vi "_API_BINANCE_GET_TickSize.vi"(0 "BinanceAPI in":refnum<class "BinanceAPI_.lvclass">, 5 "TickSize":cluster{"symbol (eg. BTCUSDT)":string}, 11 "error in (no error)":errorcluster) -> (4 "BinanceAPI out":refnum<class "BinanceAPI_.lvclass">, 6 "TickSize":dbl, 15 "error out":errorcluster)   [LabVIEW 2022 SP3, in "BinanceAPI_.lvclass"]
doc: "https://binance-docs.github.io/apidocs/spot/en/#exchange-information\n\nYou must understand what is <B>ticker size</B>"
uses:
  BinanceAPI_.lvclass
  BinanceAPI_.lvclass/BinanceAPI_.ctl
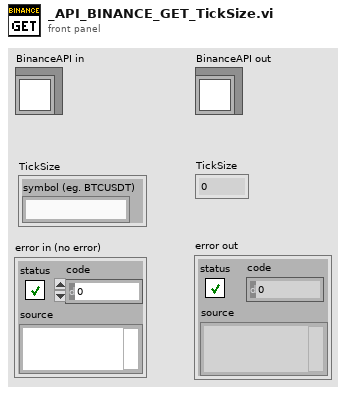
[diagram p1: front panel]
types:
  T1 = enum16{"SPOT", "USDT_FUTURES", "COIN_FUTURES", "VANILLA"}
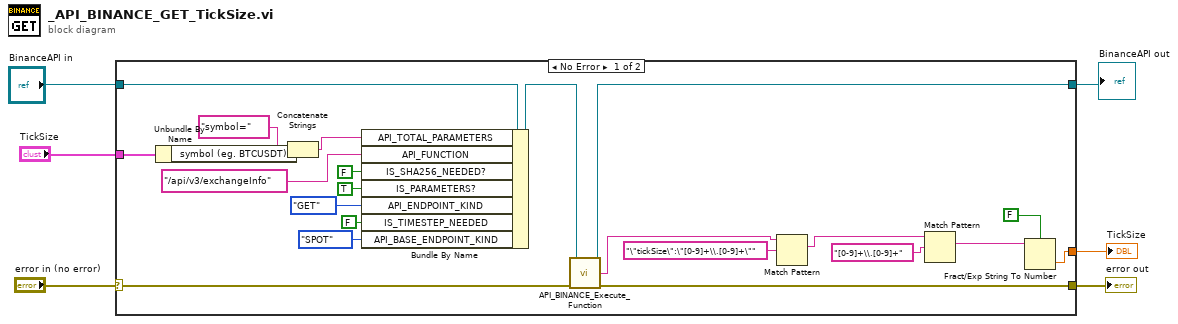
[diagram p0: block diagram]
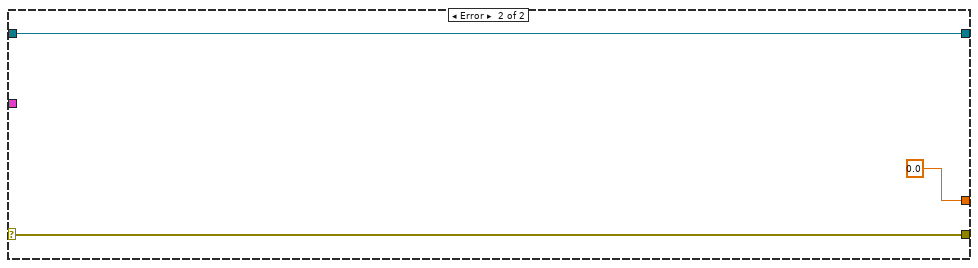
[diagram p2: hidden frame]
diagram:
  n1 = case shown="No Error" "error in (no error)" {
    selector: "error in (no error)" -> [w17 w31]
    tunnel: [w16 w31] -> w5
    tunnel: [w18 w30] -> w2
    tunnel: "BinanceAPI in" -> [w28 w30]
    tunnel: "TickSize" -> [w21 _]
    tunnel: [w9 0.0] -> w4
    frame No Error {
      n2 = Unbundle By Name(w21) -> ("symbol (eg. BTCUSDT)"=w20:string)
      n3 = Concatenate Strings("symbol=", w20) -> (w22:string)
      n4 = Bundle By Name(cluster=w28, "API_TOTAL_PARAMETERS"=w22, "API_FUNCTION"="/api/v3/exchangeInfo", "IS_SHA256_NEEDED?"=FALSE, "IS_PARAMETERS?"=TRUE, "API_ENDPOINT_KIND"=enum16{"POST", "DELETE", "GET", "PUT"}."GET", "IS_TIMESTEP_NEEDED"=FALSE, "API_BASE_ENDPOINT_KIND"=T1."SPOT") -> (w19:refnum<class "BinanceAPI_.lvclass">)
      n5 = call "API_BINANCE_Execute_Function.vi"("BinanceAPI in"=w19, "error in (no error)"=w17) -> ("BinanceAPI out"=w18:refnum<class "BinanceAPI_.lvclass">, "Body"=w13:string, "error out"=w16:errorcluster)  [unwired: 9 in, 2 out]
      n6 = Match Pattern(string=w13, regular expression="\"tickSize\":\"[0-9]+\\.[0-9]+\"") -> (match substring=w12:string)  [unwired: 1 in, 3 out]
      n7 = Match Pattern(string=w12, regular expression="[0-9]+\\.[0-9]+") -> (match substring=w10:string)  [unwired: 1 in, 3 out]
      n8 = Fract/Exp String To Number(use system decimal point (T)=FALSE, string=w10) -> (number=w9:dbl)  [unwired: 2 in, 1 out]
    }
    frame Error {
    }
  }
  "error out" <- w5
  "TickSize" <- w4
  "BinanceAPI out" <- w2
